vi "SP Find Waveform by Name.vi"(4 "error in (no error)":errorcluster, 5 "Attribute Value (\"\")":string, 6 "Attribute Name (NI_ChannelName)":string="NI_ChannelName", 7 "Results":waveform(dbl)[](array[waveform])) -> (0 "error out":errorcluster, 1 "Found Match?":bool, 2 "Waveforms":waveform(dbl)[](array[waveform]), 3 "dup Results":waveform(dbl)[](array[waveform]))   [LabVIEW 2011]
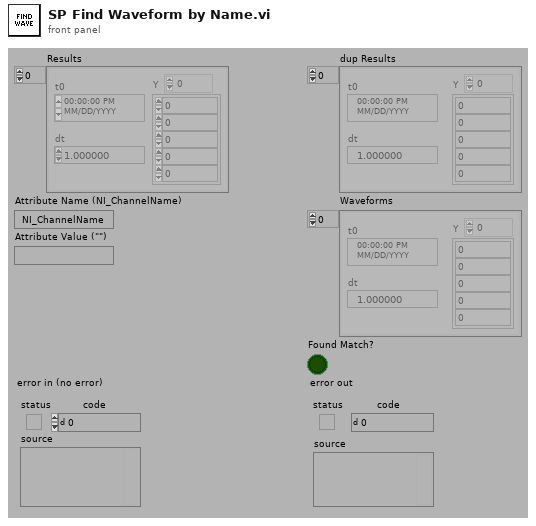
[diagram p1: front panel]
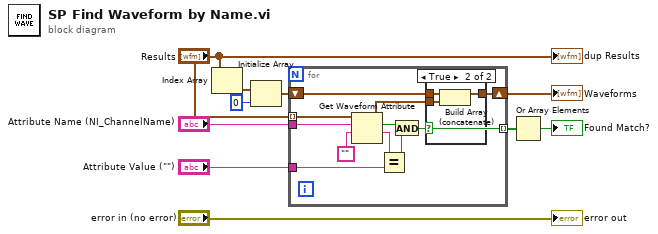
[diagram p0: block diagram]
diagram:
  n1 = Index Array(array="Results") -> (element=w3:waveform(dbl))  [unwired: 1 in]
  n2 = Initialize Array(w3, 0 ("dimension size")) -> (w2:waveform(dbl)[])
  n3 = for {
    tunnel: "Results" -> [w21] mode=indexing
    tunnel: "Attribute Value (\"\")" -> [w16]
    tunnel: "Attribute Name (NI_ChannelName)" -> [w15]
    tunnel: [w11] -> w7 mode=indexing
    shift-right: [w13] -> w5
    shift-left: w2 -> [w14]
    n4 = Get Waveform Attribute(5:"", 6:w15, 7:w21) -> (1:w18:string, 2:w19:bool, 3:w12:waveform(dbl))  [unwired: 1 in, 1 out]
    n5 = Equal?(x=w18, y=w16) -> (x = y?=w17:bool)
    n6 = And(x=w19, y=w17) -> (x .and. y?=w11:bool)
    n7 = case shown="True" w11 {
      tunnel: w14 -> [w22 w25]
      tunnel: [w22 w24] -> w13
      tunnel: w12 -> [_ w23]
      frame False {
      }
      frame True {
        n8 = Build Array (concatenate)(w25, w23) -> (w24:waveform(dbl)[])
      }
    }
  }
  "Waveforms" <- w5
  n9 = Or Array Elements(Boolean array=w7) -> (logical OR=→"Found Match?":bool)
  "dup Results" <- "Results"
  "error out" <- "error in (no error)"
